vi "Untitled 2 (SubVI).vi"(11 "Actuation Network":T2) -> (3 "Acquisition Network":T1)   [LabVIEW 2011, in "Controller VIs.lvlib"]
uses:
  Controller VIs.lvlib
  Types Definitions/Type Actuation Network Configuration.ctl
  Types Definitions/Type Acquisition Network Configuration.ctl
  Type Definitions.lvlib
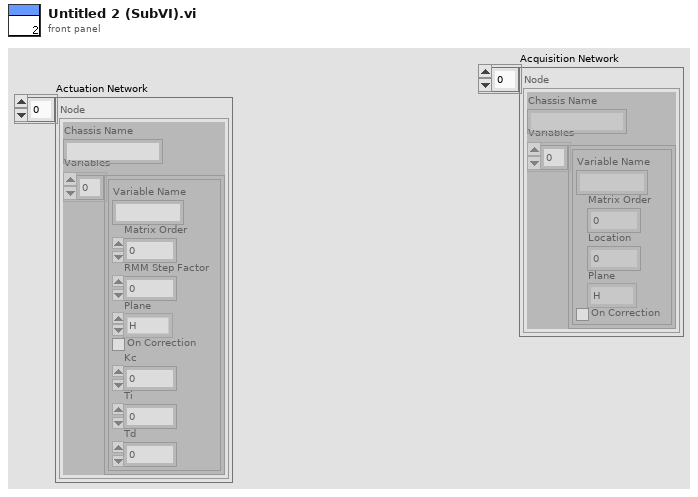
[diagram p1: front panel]
types:
  T1 = typedef "Type Definitions.lvlib/Type Acquisition Network Configuration.ctl" = cluster{"Chassis Name":string, "Variables":cluster{"Variable Name":string, "Matrix Order":u32, "Location":dbl, "Plane":enum8{"H", "V"}, "On Correction":bool}[]}[]
  T2 = typedef "Type Definitions.lvlib/Type Actuation Network Configuration.ctl" = cluster{"Chassis Name":string, "Variables":cluster{"Variable Name":string, "Matrix Order":u32, "RMM Step Factor":dbl, "Plane":enum8{"H", "V"}, "On Correction":bool, "Kc":dbl, "Ti":dbl, "Td":dbl}[]}[]
  T3 = cluster{"Chassis Name":string, "Variables":cluster{"Variable Name":string, "Matrix Order":u32, "Location":dbl, "Plane":enum8{"H", "V"}, "On Correction":bool}[]}
  T4 = cluster{"Variable Name":string, "Matrix Order":u32, "Location":dbl, "Plane":enum8{"H", "V"}, "On Correction":bool}
  T5 = cluster{"Variable Name":string, "Matrix Order":u32, "RMM Step Factor":dbl, "Plane":enum8{"H", "V"}, "On Correction":bool, "Kc":dbl, "Ti":dbl, "Td":dbl}[]
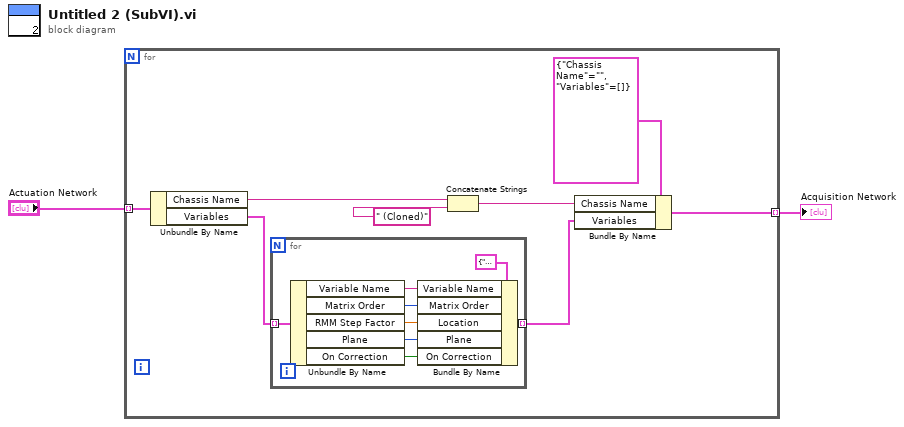
[diagram p0: block diagram]
diagram:
  n1 = for {
    tunnel: "Actuation Network" -> [w10] mode=indexing
    tunnel: [w6] -> w1 mode=indexing
    n2 = Unbundle By Name(w10) -> ("Chassis Name"=w5:string, "Variables"=w8:T5)
    n3 = for {
      tunnel: w8 -> [w18] mode=indexing
      tunnel: [w11] -> w7 mode=indexing
      n4 = Unbundle By Name(w18) -> ("Variable Name"=w16:string, "Matrix Order"=w15:u32, "RMM Step Factor"=w14:dbl, "Plane"=w13:enum8{"H", "V"}, "On Correction"=w12:bool)
      n5 = Bundle By Name(cluster=T4 {"Variable Name"="", "Matrix Order"=0, "Location"=0.0, "Plane"=enum."H", "On Correction"=FALSE} ("Variable"), "Variable Name"=w16, "Matrix Order"=w15, "Location"=w14, "Plane"=w13, "On Correction"=w12) -> (w11:T4)
    }
    n6 = Concatenate Strings(w5, " (Cloned)" ("string")) -> (w3:string)
    n7 = Bundle By Name(cluster=T3 {"Chassis Name"="", "Variables"=[]} ("Node"), "Chassis Name"=w3, "Variables"=w7) -> (w6:T3)
  }
  "Acquisition Network" <- w1
